vi "Read ADC.vi"(8 "error in (no error)":errorcluster, 10 "ADC Channel":dbl, 11 "object in":refnum<class "Cypress.lvclass">) -> (0 "error out":errorcluster, 3 "object out":refnum<class "Cypress.lvclass">)   [LabVIEW 2020, in "Cypress.lvclass"]
doc: "Read ADC es el vi donde se manda al microcontrolador los datos del canal analogico que se desea leer"
uses:
  Cypress.lvclass
  Cypress.lvclass/Cypress.ctl
  21be2342-53b6-4a26-a906-eb9eb9523aef.vi
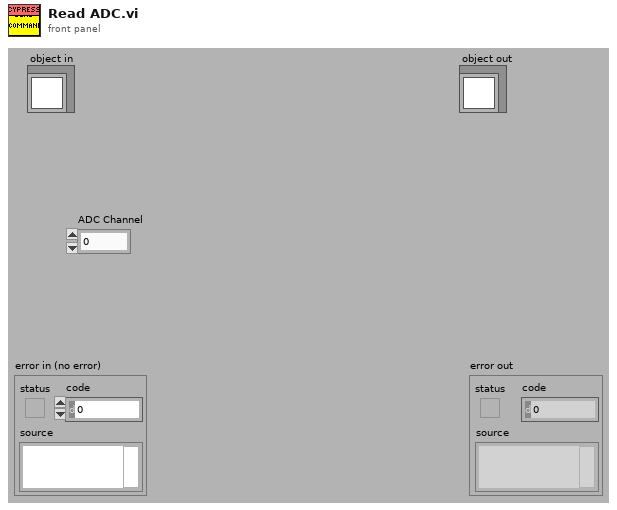
[diagram p1: front panel]
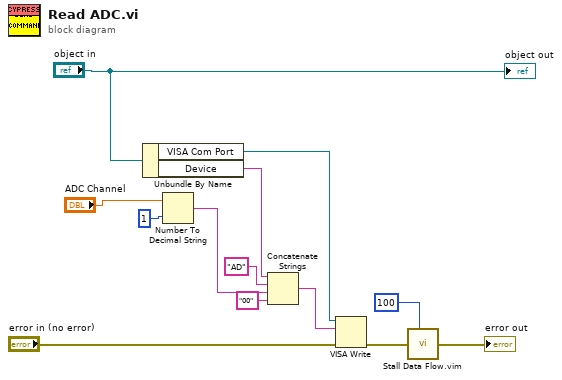
[diagram p0: block diagram]
diagram:
  n1 = Unbundle By Name("object in") -> ("VISA Com Port"=w12:refnum<visa-resource-name>, "Device"=w10:string)
  n2 = Number To Decimal String(number="ADC Channel", width (-)=i16 1) -> (decimal integer string=w9:string)
  n3 = Concatenate Strings(w10, "AD" ("string"), w9, "00" ("string")) -> (w11:string)
  n4 = VISA Write(VISA resource name=w12, write buffer=w11, error in (no error)="error in (no error)") -> (error out=w13:errorcluster)  [unwired: 2 out]
  n5 = call "Stall Data Flow.vim"("value in"=w13, "milliseconds to wait"=u32 100) -> ("value out"=→"error out":errorcluster)  [unwired: 1 out]
  "object out" <- "object in"
